vi "DestroyUserEventMessage.vi"(8 "error in":errorcluster, 11 "message ref in":refnum<class "CLM_LocalMessage_UserEvent.lvclass">) -> (0 "error out":errorcluster)   [LabVIEW 2013, in "CLM_LocalMessage_UserEvent.lvclass"]
uses:
  CLM_LocalMessage_UserEvent.lvclass
  CLM_LocalMessage_UserEvent.lvclass/CLM_LocalMessage_UserEvent.ctl
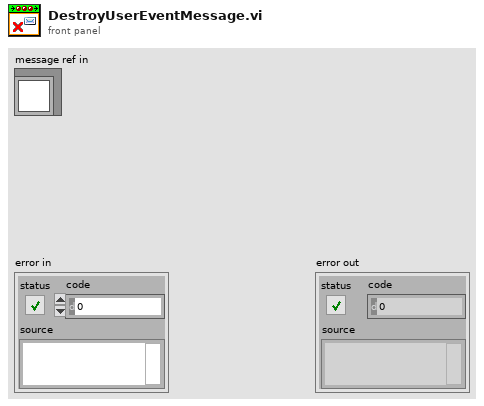
[diagram p1: front panel]
types:
  T1 = typedef "CLM_LocalMessage_UserEvent.lvclass/MessageUserEvent.ctl" = refnum<user-event>
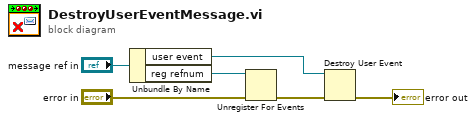
[diagram p0: block diagram]
diagram:
  n1 = Unbundle By Name("message ref in") -> ("user event"=w4:T1, "reg refnum"=w3:refnum<event-registration>)
  n2 = Unregister For Events(event registration refnum=w3, error in="error in") -> (error out=w1:errorcluster)
  n3 = Destroy User Event(user event=w4, error in=w1) -> (error out=→"error out":errorcluster)
